vi "PXIe-4139 RT Driver VI.vi"(6 "Device Clock":string, 9 "Device Inputs FIFO":refnum<k33>, 10 "Device Outputs FIFO":refnum<k33>, 11 "Device Reference":T1 format="%.0x") -> ()   [LabVIEW 2023, in "PXIe-4139 Custom Device.lvlib"]
uses:
  PXIe-4139 Custom Device.lvlib
  <vilib>/NI VeriStand/Custom Device API/Custom Device Item Ref.ctl
  <vilib>/NI VeriStand/Custom Device API/Custom Device Channel Type.ctl
  <vilib>/Platform/TimedLoop/XDataNode/timing_clust.ctl
  <vilib>/Platform/TimedLoop/XDataNode/nitl_modes.ctl
  <vilib>/Platform/TimedLoop/XDataNode/wakeup.ctl
  <vilib>/ptbypt/Other Functions.llb/Boolean Crossing PtByPt.vi
  <vilib>/Platform/TimedLoop/XDataNode/XDataNode.xnode
  <vilib>/Platform/TimedLoop/XDataNode/XDNodeRunTimeDep.lvlib
  <vilib>/NI VeriStand/Custom Device API/Custom Device API.lvlib
  <vilib>/NI VeriStand/Custom Device Tools/Custom Device Utility Library/Custom Device Utility Library.lvlib
panel:
  in  "Status Notifier":refnum<notifier>
  # "Custom Device Template\nv1.0"
  # "Use this template as a starting point for creating a custom device code module. The input controls shown here are specially named controls that the system will use to provide the device loop with data. The controls are not required for the device loop to run. For instance, if the device doesn't produce any output data, then you don't need the Device Outputs FIFO control. If you do use these controls, however, they need to have these exact names to be functional."
  # "The optional status notifier element is used to notify the RT engine of the last state of the custom device, and to indicate the device has completed execution. If this control is not used, a default No Error value is returned to the system when the device finishes execution.\n\nNote: This error state is not checked until the system shuts down. Use an output status channel to send more immediate status values to the system."
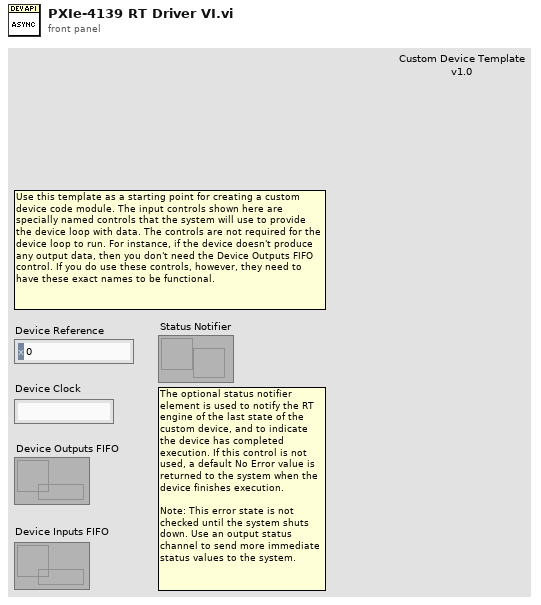
[diagram p1: front panel]
types:
  T1 = typedef "Custom Device API.lvlib/Custom Device Item Ref.ctl" = u64
  T2 = typedef "Custom Device API.lvlib/Custom Device Channel Type.ctl" = enum16{"Input", "Output"}
  T3 = typedef "Custom Device API.lvlib/Custom Device Item Info.ctl" = cluster{"Name":string, "Is Channel":bool, "GUID":string, "Is Waveform":bool}
  T4 = typedef "Custom Device API.lvlib/Custom Device Timed Loop Priority.ctl" = enum32{"Low", "Medium", "High"}
  T5 = typedef "XDNodeRunTimeDep.lvlib/timing_clust.ctl" = cluster{"Expected End [f-1]":u64, "Actual End [f-1]":u64, "Finished Late? [f-1]":bool, "Expected End [i-1]":u64, "Actual End [i-1]":u64, "Finished Late? [i-1]":bool, "Expected Start [i]":u64, "Actual Start [i]":u64, "Expected Start [f]":u64, "Actual Start [f]":u64, "Source Name":string, "Structure Name":string, "Period":i64, "Deadline":i64, "Offset":i64, "Start":i64, "Priority":i32, "Timeout":i32, "Mode":T6, "Wakeup Reason":T7, "Error":errorcluster, "Source Type":string, "Secondary Source Type":string, "Global End Time":u64, "Global Start Time":u64, "Frame Duration":u64, "Iteration Duration":u64, "Assigned CPU":i32, "I/O Scan Engine Mode":u32}
  T6 = typedef "XDNodeRunTimeDep.lvlib/nitl_modes.ctl" = enum32{"No Change", "Process missed periods, maintain original phase", "Discard missed periods, maintain original phase", "Process missed periods, ignore original phase", "Discard missed periods, ignore original phase"}
  T7 = typedef "XDNodeRunTimeDep.lvlib/wakeup.ctl" = enum32{"Normal", "Aborted", "Asynchronous wakeup", "Timing source error", "Timed loop error", "Timeout"}
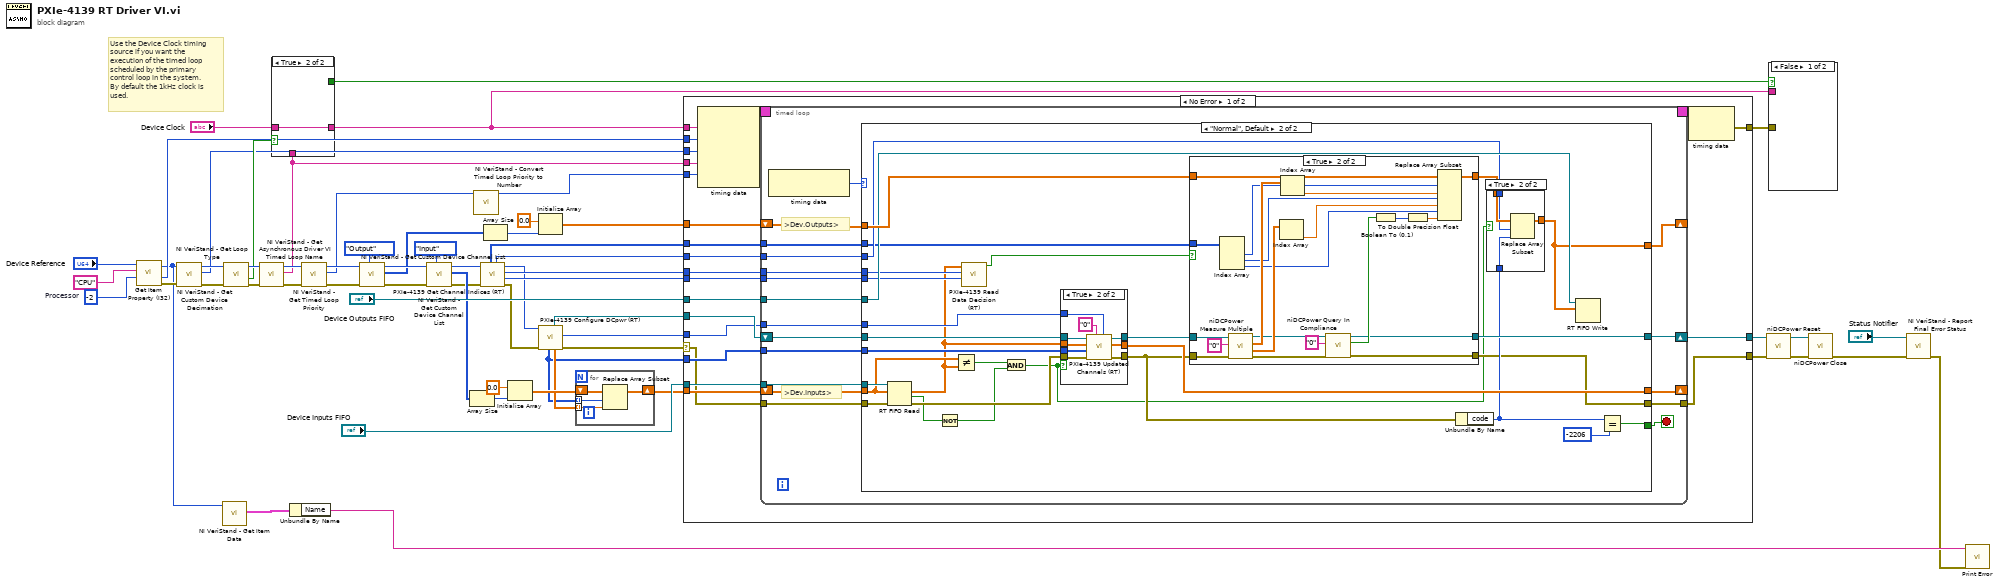
[diagram p0: block diagram]
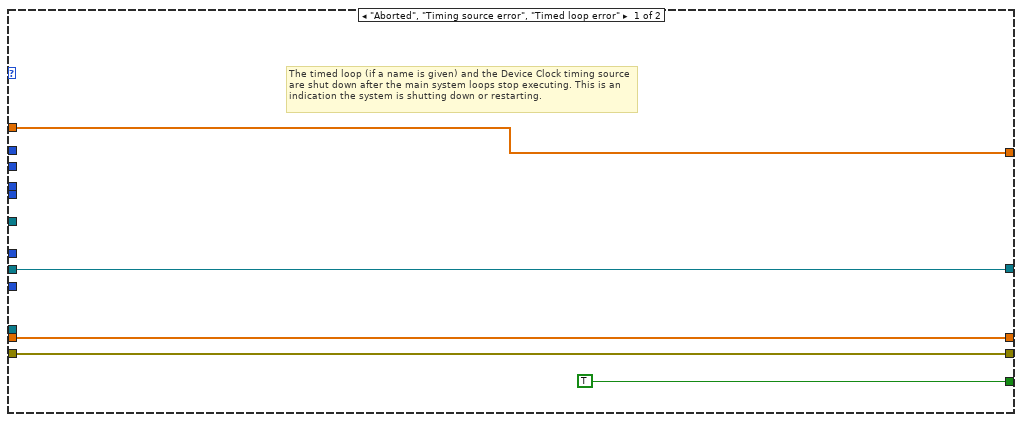
[diagram p2: hidden frame]
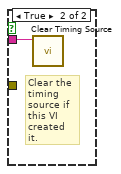
[diagram p7: hidden frame]
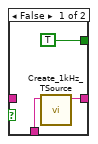
[diagram p8: hidden frame]
diagram:
  w34 = -2  # Processor
  # "Use the Device Clock timing source if you want the execution of the timed loop scheduled by the primary control loop in the system. \nBy default the 1kHz clock is used."
  n1 = call <vilib>:"Get Item Property (I32).vi"("Default Value"=w34, "Property Name"="CPU", "Item Ref in"="Device Reference") -> ("error out"=w33:errorcluster, "Value"=w28:i32, "Item Ref out"=w13:T1)  [unwired: 5 in, 1 out]
  n2 = call <vilib>:"NI VeriStand - Get Custom Device Decimation.vi"("error in (no error)"=w33, "Device Ref in"=w13) -> ("error out"=w30:errorcluster, "Decimation"=w29:i32, "Device Ref out"=w31:T1)  [unwired: 7 in]
  n3 = call <vilib>:"NI VeriStand - Get Item Data.vi"("Item Ref in"=w13) -> ("Item Info"=w12:T3)  [unwired: 7 in, 3 out]
  n4 = call <vilib>:"NI VeriStand - Get Loop Type.vi"("error in (no error)"=w30, "Device Ref in"=w31) -> ("error out"=w43:errorcluster, "Use Device Clock"=w41:bool, "Device Ref out"=w42:T1)  [unwired: 7 out]
  n5 = call <vilib>:"NI VeriStand - Get Asynchronous Driver VI Timed Loop Name.vi"("error in (no error)"=w43, "Device Ref in"=w42) -> ("error out"=w48:errorcluster, "Device Timed Loop Name"=w35:string, "Device Ref out"=w60:T1)  [unwired: 7 out]
  n6 = case shown="True" w41 {
    tunnel: "Device Clock" -> [_ w64]
    tunnel: [w63 w64] -> w36
    tunnel: [TRUE _] -> w37
    tunnel: w35 -> [w61 _]
    frame False {
      n7 = call <vilib>:"Create_1kHz_TSource.vi"("name (in)"=w61) -> ("name (out)"=w63:string)  [unwired: 1 in, 9 out]
    }
    frame True {
    }
  }
  n8 = Unbundle By Name(w12) -> ("Name"=w11:string)
  n9 = call <vilib>:"NI VeriStand - Get Timed Loop Priority.vi"("error in (no error)"=w48, "Device Ref in"=w60) -> ("error out"=w49:errorcluster, "Priority"=w46:T4, "Device Ref out"=w50:T1)  [unwired: 7 out]
  n10 = call <vilib>:"NI VeriStand - Get Custom Device Channel List.vi"("Channel Type"=Custom_Device_Channel_Type."Output", "error in (no error)"=w49, "Device Ref in"=w50) -> ("error out"=w52:errorcluster, "Specified Channel Ref List"=w47:T1[], "Device Ref out"=w53:T1)  [unwired: 6 out]
  n11 = call <vilib>:"NI VeriStand - Get Custom Device Channel List.vi"("Channel Type"=Custom_Device_Channel_Type."Input", "error in (no error)"=w52, "Device Ref in"=w53) -> ("error out"=w20:errorcluster, "Specified Channel Ref List"=w21:T1[], "Device Ref out"=w22:T1)  [unwired: 6 out]
  n12 = Array Size(array=w21) -> (size(s)=w44:i32)
  n13 = call <vilib>:"NI VeriStand - Convert Timed Loop Priority to Number.vi"("Priority"=w46) -> ("Numeric Priority"=w45:i32)  [unwired: 10 out]
  n14 = call "PXIe-4139 Get Channel Indices (RT).vi"("error in (no error)"=w20, "Device Item Ref In"=w22) -> ("error out"=w17:errorcluster, "Read Trigger Index"=w18:i32, "Continuous Read? Index"=w19:i32, "Device Item Ref Out"=w16:T1, "error index"=w4:i32, "channel output FIFO indexes"=w3:i32[])  [unwired: 4 in]
  n15 = Array Size(array=w47) -> (size(s)=w2:i32)
  n16 = Initialize Array(0.0 ("element"), w44) -> (w8:dbl[])
  n17 = Initialize Array(0.0 ("element"), w2) -> (w55:dbl[])
  n18 = call "PXIe-4139 Configure DCpwr (RT).vi"("error in (no error)"=w17, "Device Ref in"=w16) -> ("error out"=w1:errorcluster, "Channel 0 Type"=w9:i32, "Defaults"=w6:dbl[], "instrument handle out"=w15:refnum<k15>, "input FIFO Indexes"=w5:i32[])  [unwired: 4 in, 1 out]
  n19 = for {
    shift-right: [w67] -> w7
    shift-left: w8 -> [w68]
    tunnel: w5 -> [w66] mode=indexing
    tunnel: w6 -> [w65] mode=indexing
    n20 = Replace Array Subset(array=w68, new element=w65, index=w66) -> (w67:dbl[])
  }
  n21 = case shown="No Error" w1 {
    selector: w1 -> [w71 w197]
    tunnel: "Device Outputs FIFO" -> [w88 _]
    tunnel: "Device Inputs FIFO" -> [w87 _]
    tunnel: w55 -> [w86 _]
    tunnel: w45 -> [w85 _]
    tunnel: [w84 _] -> w38
    tunnel: w36 -> [w83 _]
    tunnel: w35 -> [w82 _]
    tunnel: w29 -> [w81 _]
    tunnel: w28 -> [w80 _]
    tunnel: [w79 w196] -> w25
    tunnel: [w78 w197] -> w24
    tunnel: w19 -> [w77 _]
    tunnel: w18 -> [w76 _]
    tunnel: w15 -> [w75 w196]
    tunnel: w9 -> [w74 _]
    tunnel: w7 -> [w73 _]
    tunnel: w5 -> [w72 _]
    tunnel: w4 -> [w70 _]
    tunnel: w3 -> [w69 _]
    frame No Error {
      n22 = node-c288(w83, w80, w81, w82, w85) -> (w90:T5)
      n23 = timed-loop {
        timing: w90 -> [_]
        timing-out: [_] -> w89
        shift-right: [w106] -> _
        shift-left: w73 -> [w107]
        shift-right: [w103] -> _
        shift-left: w86 -> [w104]
        tunnel: w88 -> [w102]
        tunnel: w87 -> [w101]
        shift-right: [w98] -> w79
        shift-left: w75 -> [w99]
        tunnel: w77 -> [w97]
        tunnel: w76 -> [w96]
        tunnel: w74 -> [w95]
        tunnel: w72 -> [w94]
        tunnel: w70 -> [w92]
        tunnel: w71 -> [w108]
        tunnel: [w100] -> w78
        tunnel: w69 -> [w91]
        stop <- w93 stop-if-true
        # ">Dev.Outputs>"
        # ">Dev.Inputs>"
        n24 = node-c288() -> (w105:T7)  [unwired: 1 out]
        n25 = case shown="\"Normal\", Default" w105 {
          tunnel: w108 -> [w112 w141]
          tunnel: w107 -> [w113 w126]
          tunnel: [w112 w116] -> w100
          tunnel: [w113 w136] -> w106
          tunnel: w104 -> [w111 w140]
          tunnel: [w111 w120] -> w103
          tunnel: w102 -> [_ w139]
          tunnel: w101 -> [_ w142]
          tunnel: [TRUE w122] -> w93
          tunnel: w99 -> [w109 w138]
          tunnel: [w109 w134] -> w98
          tunnel: w97 -> [_ w133]
          tunnel: w96 -> [_ w132]
          tunnel: w95 -> [_ w130]
          tunnel: w94 -> [_ w127]
          tunnel: w92 -> [_ w119]
          tunnel: w91 -> [_ w117]
          frame "Aborted", "Timing source error", "Timed loop error" {
            # "The timed loop (if a name is given) and the Device Clock timing source are shut down after the main system loops stop executing. This is an indication the system is shutting down or restarting."
          }
          frame "Normal", Default {
            n26 = RT FIFO Read(0:w142, 1:w126, 3:w141) -> (9:w125:dbl[], 10:w129:bool, 11:w135:errorcluster)  [unwired: 3 out]
            n27 = Not(x=w129) -> (.not. x?=w128:bool)
            n28 = Not Equal?(x=w126, y=w125) -> (x != y?=w124:bool)
            n29 = call "PXIe-4139 Read Data Decision (RT).vi"("Read Trigger Index"=w132, "Continuous Read? Index"=w133, "Array In"=w125) -> ("Read Data?"=w131:bool)  [unwired: 8 in]
            n30 = And(x=w124, y=w128) -> (x .and. y?=w114:bool)
            n31 = case shown="True" w114 {
              tunnel: w138 -> [w173 w183]
              tunnel: [w173 w180] -> w137
              tunnel: [w174 w181] -> w136
              tunnel: [w172 w179] -> w115
              tunnel: w135 -> [w172 w178]
              tunnel: w125 -> [w174 w182]
              tunnel: w130 -> [_ w176]
              tunnel: w127 -> [_ w175]
              frame False {
              }
              frame True {
                n32 = call "PXIe-4139 Updated Channels (RT).vi"("Channel Type"=w176, "Channel"="0", "error in (no error)"=w178, "FIFO Indexes"=w175, "Data In"=w182, "resource name In"=w183) -> ("error out"=w179:errorcluster, "Data Out"=w181:dbl[], "resource name Out"=w180:refnum<k15>)  [unwired: 3 in]
              }
            }
            n33 = case shown="True" w131 {
              tunnel: [w150 w171] -> w121
              tunnel: w140 -> [w150 w170]
              tunnel: w137 -> [w149 w156]
              tunnel: w115 -> [w148 w155]
              tunnel: [w148 w161] -> w116
              tunnel: [w149 w162] -> w134
              tunnel: w117 -> [_ w154]
              frame False {
              }
              frame True {
                n34 = Index Array(array=w154) -> (element #1=w153:i32, element #2=w152:i32, element #3=w151:i32)  [unwired: 3 in]
                n35 = call <instrlib>:"niDCPower Measure Multiple.vi"("error in (no error)"=w155, "channel name"="0", "instrument handle"=w156) -> ("error out"=w157:errorcluster, "current measurements"=w168:dbl[], "voltage measurements"=w169:dbl[], "instrument handle out"=w158:refnum<k15>)  [unwired: 5 in]
                n36 = Index Array(array=w168) -> (element=w163:dbl)  [unwired: 1 in]
                n37 = Index Array(array=w169) -> (element=w167:dbl)  [unwired: 1 in]
                n38 = call <instrlib>:"niDCPower Query In Compliance.vi"("error in (no error)"=w157, "channel name"="0", "instrument handle"=w158) -> ("error out"=w161:errorcluster, "in compliance?"=w166:bool, "instrument handle out"=w162:refnum<k15>)  [unwired: 6 in]
                n39 = Boolean To (0,1)(Boolean=w166) -> (0, 1=w165:i16)
                n40 = To Double Precision Float(number=w165) -> (double precision float=w164:dbl)
                n41 = Replace Array Subset(array=w170, new element #1=w167, index #1=w153, new element #2=w163, index #2=w152, new element #3=w164, index #3=w151) -> (w171:dbl[])
              }
            }
            n42 = Unbundle By Name(w115) -> ("code"=w118:i32)
            n43 = case shown="True" w114 {
              tunnel: w121 -> [w143 w147]
              tunnel: [w143 w146] -> w120
              tunnel: w119 -> [_ w145]
              tunnel: w118 -> [_ w144]
              frame False {
              }
              frame True {
                n44 = Replace Array Subset(array=w147, new element=w144, index=w145) -> (w146:dbl[])
              }
            }
            n45 = RT FIFO Write(0:w139, 1:w120) -> ()  [unwired: 2 in, 5 out]
            n46 = Equal?(x=w118, y=-2206) -> (x = y?=w122:bool)
          }
        }
      }
      n47 = node-c288(w89) -> (w84:errorcluster)
    }
    frame Error {
    }
  }
  n48 = call <instrlib>:"niDCPower Reset.vi"("error in (no error)"=w24, "instrument handle"=w25) -> ("error out"=w27:errorcluster, "instrument handle out"=w26:refnum<k15>)  [unwired: 8 in]
  n49 = case shown="False" w37 {
    tunnel: w38 -> [_ _]
    tunnel: w36 -> [_ w198]
    frame False {
    }
    frame True {
      # "Clear the timing source if this VI created it."
      n50 = call <vilib>:"Clear Timing Source.vi"("name"=w198) -> ()  [unwired: 1 in, 10 out]
    }
  }
  n51 = call <instrlib>:"niDCPower Close.vi"("error in (no error)"=w27, "instrument handle"=w26) -> ("error out"=w14:errorcluster)  [unwired: 9 in]
  n52 = call <vilib>:"NI VeriStand - Report Final Error Status.vi"("error in (no error)"=w14, "Status Notifier"="Status Notifier") -> ("error out"=w10:errorcluster)  [unwired: 1 in, 8 out]
  n53 = call "Print Error.vi"("error out"=w10, "Your code's public name"=w11) -> ()  [unwired: 9 in]
